vi "OPEN VALVE in Corect Direction.vi"(4 "time after close":u32, 6 "Valve DIR":T1, 7 "changed or first call?":bool, 8 "error in (no error)":errorcluster, 11 "Stand in":refnum<class "Stand.lvclass">) -> (0 "error out":errorcluster, 2 "Done":bool, 3 "Stand out":refnum<class "Stand.lvclass">)   [LabVIEW 2019, in "Stand.lvclass"]
uses:
  Stand.lvclass
  C:/Users/ANENKOV_V1/Desktop/src/Device_class/Device.lvclass
  Valve DIR.ctl
  Device_class/Device.lvclass/Device.ctl
  FPGA/TypeDef/DO index.ctl
  DoValve.vi/e7d2c9dc-ba67-4685-b926-bcce34aa2778.vi
  DoValve.vi/628819af-fd07-4303-9780-3ddd467101db.vi
  Const All Valve.vi
  FPGA_API_class/FPGA API.lvclass
  Device_class/Device.lvclass
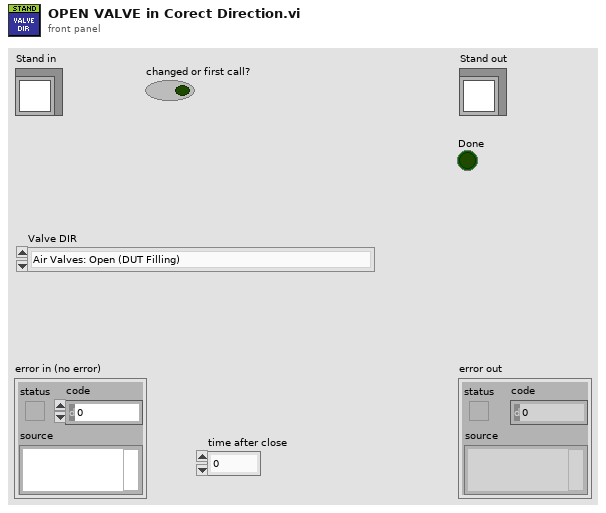
[diagram p1: front panel]
types:
  T1 = typedef "Valve DIR.ctl" = enum16{"Air Valves: Open (DUT Filling)", "Air Valves: Open (Chamber Filling)", "Air Valves: Open (Pump Pressure DUT)", "Air Valves: Open (Pump Pressure Chamber)", "Air Valves: Open (Haskel Pressure DUT)", "Air Valves: Open (Haskel Pressure Chamber)", "Air Valves: Open (Slow Release DUT)", "Air Valves: Open (Slow Release Chamber)", "Air Valves: Open (Fast Release DUT)", "Air Valves: Open (Fast Release Chamber)", "Air Valves: Open (Emergency Release DUT and Chamber)", "Air Valves: Leak Hi (Chamber)", "Air Valves: Leak Hi (DUT)", "Air Valves: Backpressure (Chamber)", "Air Valves: Backpressure (DUT)", "Air Valves: Fully Closed", "Air Valves: Open 33.7"}
  T2 = typedef "DO index.ctl" = u8
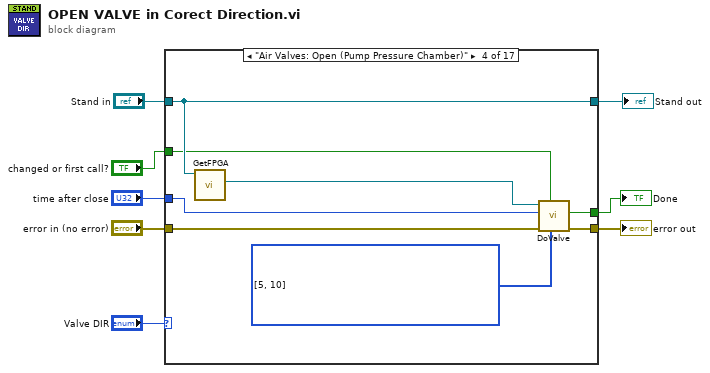
[diagram p0: block diagram]
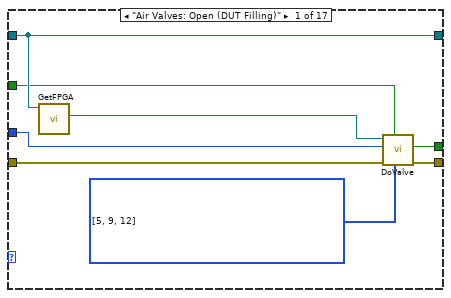
[diagram p2: hidden frame]
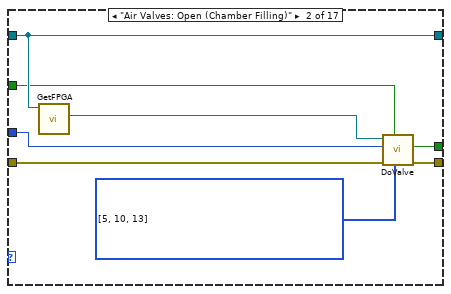
[diagram p3: hidden frame]
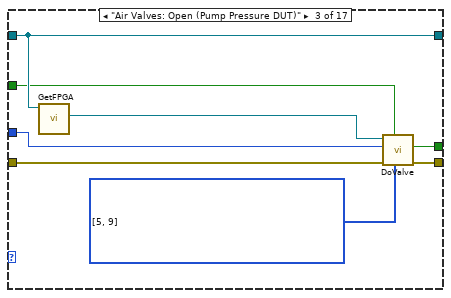
[diagram p4: hidden frame]
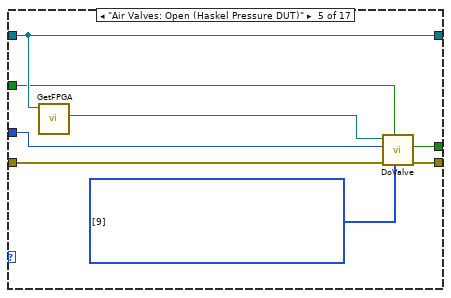
[diagram p5: hidden frame]
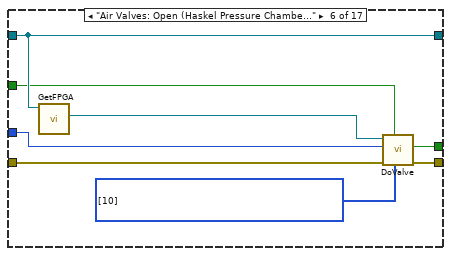
[diagram p6: hidden frame]
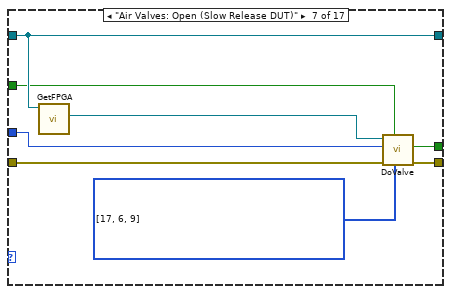
[diagram p7: hidden frame]
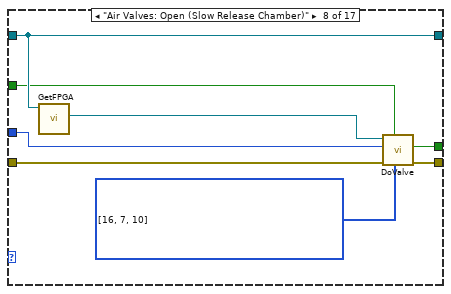
[diagram p8: hidden frame]
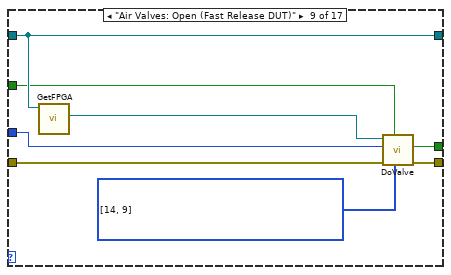
[diagram p9: hidden frame]
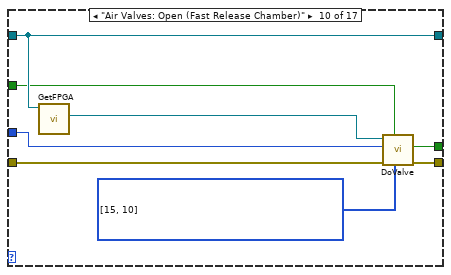
[diagram p10: hidden frame]
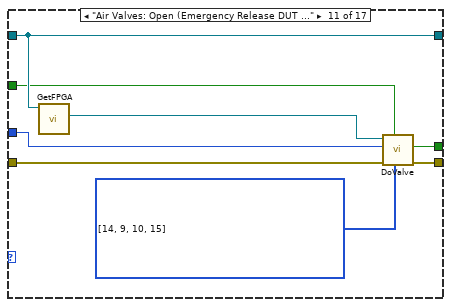
[diagram p11: hidden frame]
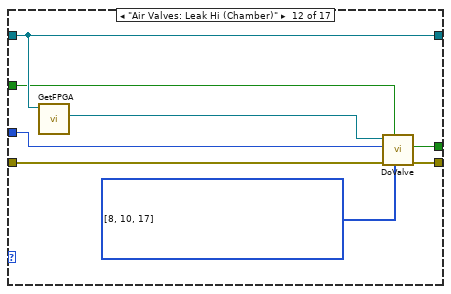
[diagram p12: hidden frame]
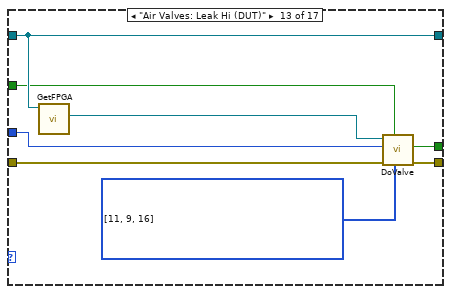
[diagram p13: hidden frame]
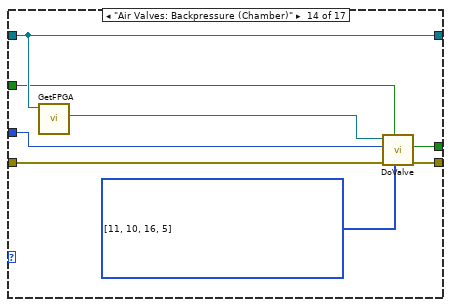
[diagram p14: hidden frame]
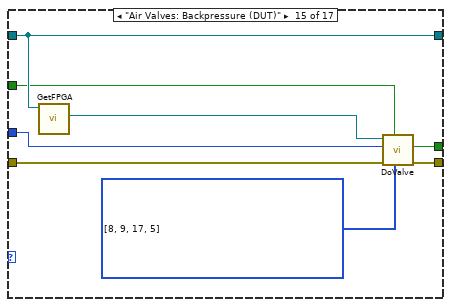
[diagram p15: hidden frame]
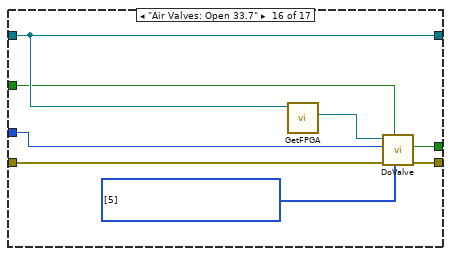
[diagram p16: hidden frame]
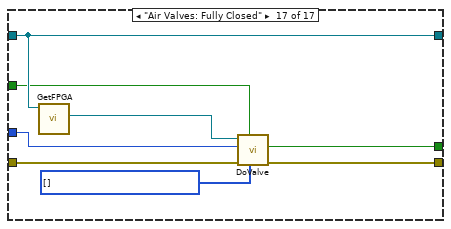
[diagram p17: hidden frame]
diagram:
  n1 = case shown="\"Air Valves: Open (Pump Pressure Chamber)\"" "Valve DIR" {
    tunnel: [w16 w24 w32 w40 w48 w56 w64 w72 w80 w88 w96 w104 w112 w120 w128 w136 w144] -> w3
    tunnel: "Stand in" -> [w16 w24 w32 w40 w48 w56 w64 w72 w80 w88 w96 w104 w112 w120 w128 w136 w144]
    tunnel: [w12 w21 w29 w37 w45 w53 w61 w69 w77 w85 w93 w101 w109 w117 w125 w133 w141] -> w8
    tunnel: "error in (no error)" -> [w14 w22 w30 w38 w46 w54 w62 w70 w78 w86 w94 w102 w110 w118 w126 w134 w142]
    tunnel: [w10 w18 w26 w34 w42 w50 w58 w66 w74 w83 w90 w98 w106 w114 w122 w130 w138] -> w2
    tunnel: "changed or first call?" -> [w11 w19 w27 w35 w43 w51 w59 w67 w75 w82 w91 w99 w107 w115 w123 w131 w139]
    tunnel: "time after close" -> [w9 w17 w25 w33 w41 w49 w57 w65 w73 w81 w89 w97 w105 w113 w121 w129 w137]
    frame "Air Valves: Open (DUT Filling)" {
      w13 = T2[] [5, 9, 12] items=["DO 0 [KP1] [M12]", "DO 1 [ON KP2] [M21]", "DO 2 [ON KP3] [M24]", "DO 3 [WATER Y18.1 [DO3]]", "DO 4 [WATER Y18.2 [DO4]]", "DO 5 [KP6 Y29.1 33.7]", "DO 6 [KP7 Y29.2 33.8]", "DO 7 [KP8 Y29.3 33.9]", "DO 8 [KP9 Y29.4  33.12]", "DO 9 [KP10 Y29.5 33.1]", "DO 10 [KP11 Y29.6 33.2]", "DO 11 [KP12 Y29.7  33.13]", "DO 12 [KP13 Y29.8  33.11]", "DO 13 [KP14 Y29.9 33.10]", "DO 14 [KP15 Y29.10  33.6]", "DO 15 [KP16 Y29.11  33.5]", "DO 16 [KP17 Y29.12  33.4]", "DO 17 [KP18 Y29.13 33.3]", "DO 18 [AIR KP19]", "DO 19 [STEP DRIVE EN KP20]", "DO 20 [KP21 Y44.1 OPEN]", "DO 21 [ KP22 Y44.1 CLOSE]", "DO 22 [ KP23 Y44.2 OPEN]", "DO 23", "DO 24 [STEP DRIVE 1]", "DO 25 [STEP DRIVE 2]"] ("#DO")
      n2 = call "GetFPGA.vi"("Device in"=w16) -> ("FPGA API.lvclass"=w15:refnum<class "FPGA API.lvclass">)  [unwired: 10 in]
      n3 = call "DoValve.vi"("#DO"=w13, "Reset"=w11, "error in (no error)"=w14, "time after close"=w9, "reference in"=w15) -> ("error out"=w12:errorcluster, "Done"=w10:bool)  [unwired: 4 in, 1 out]
    }
    frame "Air Valves: Open (Chamber Filling)" {
      w20 = T2[] [5, 10, 13] items=["DO 0 [KP1] [M12]", "DO 1 [ON KP2] [M21]", "DO 2 [ON KP3] [M24]", "DO 3 [WATER Y18.1 [DO3]]", "DO 4 [WATER Y18.2 [DO4]]", "DO 5 [KP6 Y29.1 33.7]", "DO 6 [KP7 Y29.2 33.8]", "DO 7 [KP8 Y29.3 33.9]", "DO 8 [KP9 Y29.4  33.12]", "DO 9 [KP10 Y29.5 33.1]", "DO 10 [KP11 Y29.6 33.2]", "DO 11 [KP12 Y29.7  33.13]", "DO 12 [KP13 Y29.8  33.11]", "DO 13 [KP14 Y29.9 33.10]", "DO 14 [KP15 Y29.10  33.6]", "DO 15 [KP16 Y29.11  33.5]", "DO 16 [KP17 Y29.12  33.4]", "DO 17 [KP18 Y29.13 33.3]", "DO 18 [AIR KP19]", "DO 19 [STEP DRIVE EN KP20]", "DO 20 [KP21 Y44.1 OPEN]", "DO 21 [ KP22 Y44.1 CLOSE]", "DO 22 [ KP23 Y44.2 OPEN]", "DO 23", "DO 24 [STEP DRIVE 1]", "DO 25 [STEP DRIVE 2]"] ("#DO")
      n4 = call "GetFPGA.vi"("Device in"=w24) -> ("FPGA API.lvclass"=w23:refnum<class "FPGA API.lvclass">)  [unwired: 10 in]
      n5 = call "DoValve.vi"("#DO"=w20, "Reset"=w19, "error in (no error)"=w22, "time after close"=w17, "reference in"=w23) -> ("error out"=w21:errorcluster, "Done"=w18:bool)  [unwired: 4 in, 1 out]
    }
    frame "Air Valves: Open (Pump Pressure DUT)" {
      w28 = T2[] [5, 9] items=["DO 0 [KP1] [M12]", "DO 1 [ON KP2] [M21]", "DO 2 [ON KP3] [M24]", "DO 3 [WATER Y18.1 [DO3]]", "DO 4 [WATER Y18.2 [DO4]]", "DO 5 [KP6 Y29.1 33.7]", "DO 6 [KP7 Y29.2 33.8]", "DO 7 [KP8 Y29.3 33.9]", "DO 8 [KP9 Y29.4  33.12]", "DO 9 [KP10 Y29.5 33.1]", "DO 10 [KP11 Y29.6 33.2]", "DO 11 [KP12 Y29.7  33.13]", "DO 12 [KP13 Y29.8  33.11]", "DO 13 [KP14 Y29.9 33.10]", "DO 14 [KP15 Y29.10  33.6]", "DO 15 [KP16 Y29.11  33.5]", "DO 16 [KP17 Y29.12  33.4]", "DO 17 [KP18 Y29.13 33.3]", "DO 18 [AIR KP19]", "DO 19 [STEP DRIVE EN KP20]", "DO 20 [KP21 Y44.1 OPEN]", "DO 21 [ KP22 Y44.1 CLOSE]", "DO 22 [ KP23 Y44.2 OPEN]", "DO 23", "DO 24 [STEP DRIVE 1]", "DO 25 [STEP DRIVE 2]"] ("#DO")
      n6 = call "GetFPGA.vi"("Device in"=w32) -> ("FPGA API.lvclass"=w31:refnum<class "FPGA API.lvclass">)  [unwired: 10 in]
      n7 = call "DoValve.vi"("#DO"=w28, "Reset"=w27, "error in (no error)"=w30, "time after close"=w25, "reference in"=w31) -> ("error out"=w29:errorcluster, "Done"=w26:bool)  [unwired: 4 in, 1 out]
    }
    frame "Air Valves: Open (Pump Pressure Chamber)" {
      w36 = T2[] [5, 10] items=["DO 0 [KP1] [M12]", "DO 1 [ON KP2] [M21]", "DO 2 [ON KP3] [M24]", "DO 3 [WATER Y18.1 [DO3]]", "DO 4 [WATER Y18.2 [DO4]]", "DO 5 [KP6 Y29.1 33.7]", "DO 6 [KP7 Y29.2 33.8]", "DO 7 [KP8 Y29.3 33.9]", "DO 8 [KP9 Y29.4  33.12]", "DO 9 [KP10 Y29.5 33.1]", "DO 10 [KP11 Y29.6 33.2]", "DO 11 [KP12 Y29.7  33.13]", "DO 12 [KP13 Y29.8  33.11]", "DO 13 [KP14 Y29.9 33.10]", "DO 14 [KP15 Y29.10  33.6]", "DO 15 [KP16 Y29.11  33.5]", "DO 16 [KP17 Y29.12  33.4]", "DO 17 [KP18 Y29.13 33.3]", "DO 18 [AIR KP19]", "DO 19 [STEP DRIVE EN KP20]", "DO 20 [KP21 Y44.1 OPEN]", "DO 21 [ KP22 Y44.1 CLOSE]", "DO 22 [ KP23 Y44.2 OPEN]", "DO 23", "DO 24 [STEP DRIVE 1]", "DO 25 [STEP DRIVE 2]"] ("#DO")
      n8 = call "GetFPGA.vi"("Device in"=w40) -> ("FPGA API.lvclass"=w39:refnum<class "FPGA API.lvclass">)  [unwired: 10 in]
      n9 = call "DoValve.vi"("#DO"=w36, "Reset"=w35, "error in (no error)"=w38, "time after close"=w33, "reference in"=w39) -> ("error out"=w37:errorcluster, "Done"=w34:bool)  [unwired: 4 in, 1 out]
    }
    frame "Air Valves: Open (Haskel Pressure DUT)" {
      w44 = T2[] [9] items=["DO 0 [KP1] [M12]", "DO 1 [ON KP2] [M21]", "DO 2 [ON KP3] [M24]", "DO 3 [WATER Y18.1 [DO3]]", "DO 4 [WATER Y18.2 [DO4]]", "DO 5 [KP6 Y29.1 33.7]", "DO 6 [KP7 Y29.2 33.8]", "DO 7 [KP8 Y29.3 33.9]", "DO 8 [KP9 Y29.4  33.12]", "DO 9 [KP10 Y29.5 33.1]", "DO 10 [KP11 Y29.6 33.2]", "DO 11 [KP12 Y29.7  33.13]", "DO 12 [KP13 Y29.8  33.11]", "DO 13 [KP14 Y29.9 33.10]", "DO 14 [KP15 Y29.10  33.6]", "DO 15 [KP16 Y29.11  33.5]", "DO 16 [KP17 Y29.12  33.4]", "DO 17 [KP18 Y29.13 33.3]", "DO 18 [AIR KP19]", "DO 19 [STEP DRIVE EN KP20]", "DO 20 [KP21 Y44.1 OPEN]", "DO 21 [ KP22 Y44.1 CLOSE]", "DO 22 [ KP23 Y44.2 OPEN]", "DO 23", "DO 24 [STEP DRIVE 1]", "DO 25 [STEP DRIVE 2]"] ("#DO")
      n10 = call "GetFPGA.vi"("Device in"=w48) -> ("FPGA API.lvclass"=w47:refnum<class "FPGA API.lvclass">)  [unwired: 10 in]
      n11 = call "DoValve.vi"("#DO"=w44, "Reset"=w43, "error in (no error)"=w46, "time after close"=w41, "reference in"=w47) -> ("error out"=w45:errorcluster, "Done"=w42:bool)  [unwired: 4 in, 1 out]
    }
    frame "Air Valves: Open (Haskel Pressure Chamber)" {
      w52 = T2[] [10] items=["DO 0 [KP1] [M12]", "DO 1 [ON KP2] [M21]", "DO 2 [ON KP3] [M24]", "DO 3 [WATER Y18.1 [DO3]]", "DO 4 [WATER Y18.2 [DO4]]", "DO 5 [KP6 Y29.1 33.7]", "DO 6 [KP7 Y29.2 33.8]", "DO 7 [KP8 Y29.3 33.9]", "DO 8 [KP9 Y29.4  33.12]", "DO 9 [KP10 Y29.5 33.1]", "DO 10 [KP11 Y29.6 33.2]", "DO 11 [KP12 Y29.7  33.13]", "DO 12 [KP13 Y29.8  33.11]", "DO 13 [KP14 Y29.9 33.10]", "DO 14 [KP15 Y29.10  33.6]", "DO 15 [KP16 Y29.11  33.5]", "DO 16 [KP17 Y29.12  33.4]", "DO 17 [KP18 Y29.13 33.3]", "DO 18 [AIR KP19]", "DO 19 [STEP DRIVE EN KP20]", "DO 20 [KP21 Y44.1 OPEN]", "DO 21 [ KP22 Y44.1 CLOSE]", "DO 22 [ KP23 Y44.2 OPEN]", "DO 23", "DO 24 [STEP DRIVE 1]", "DO 25 [STEP DRIVE 2]"] ("#DO")
      n12 = call "GetFPGA.vi"("Device in"=w56) -> ("FPGA API.lvclass"=w55:refnum<class "FPGA API.lvclass">)  [unwired: 10 in]
      n13 = call "DoValve.vi"("#DO"=w52, "Reset"=w51, "error in (no error)"=w54, "time after close"=w49, "reference in"=w55) -> ("error out"=w53:errorcluster, "Done"=w50:bool)  [unwired: 4 in, 1 out]
    }
    frame "Air Valves: Open (Slow Release DUT)" {
      w60 = T2[] [17, 6, 9] items=["DO 0 [KP1] [M12]", "DO 1 [ON KP2] [M21]", "DO 2 [ON KP3] [M24]", "DO 3 [WATER Y18.1 [DO3]]", "DO 4 [WATER Y18.2 [DO4]]", "DO 5 [KP6 Y29.1 33.7]", "DO 6 [KP7 Y29.2 33.8]", "DO 7 [KP8 Y29.3 33.9]", "DO 8 [KP9 Y29.4  33.12]", "DO 9 [KP10 Y29.5 33.1]", "DO 10 [KP11 Y29.6 33.2]", "DO 11 [KP12 Y29.7  33.13]", "DO 12 [KP13 Y29.8  33.11]", "DO 13 [KP14 Y29.9 33.10]", "DO 14 [KP15 Y29.10  33.6]", "DO 15 [KP16 Y29.11  33.5]", "DO 16 [KP17 Y29.12  33.4]", "DO 17 [KP18 Y29.13 33.3]", "DO 18 [AIR KP19]", "DO 19 [STEP DRIVE EN KP20]", "DO 20 [KP21 Y44.1 OPEN]", "DO 21 [ KP22 Y44.1 CLOSE]", "DO 22 [ KP23 Y44.2 OPEN]", "DO 23", "DO 24 [STEP DRIVE 1]", "DO 25 [STEP DRIVE 2]"] ("#DO")
      n14 = call "GetFPGA.vi"("Device in"=w64) -> ("FPGA API.lvclass"=w63:refnum<class "FPGA API.lvclass">)  [unwired: 10 in]
      n15 = call "DoValve.vi"("#DO"=w60, "Reset"=w59, "error in (no error)"=w62, "time after close"=w57, "reference in"=w63) -> ("error out"=w61:errorcluster, "Done"=w58:bool)  [unwired: 4 in, 1 out]
    }
    frame "Air Valves: Open (Slow Release Chamber)" {
      w68 = T2[] [16, 7, 10] items=["DO 0 [KP1] [M12]", "DO 1 [ON KP2] [M21]", "DO 2 [ON KP3] [M24]", "DO 3 [WATER Y18.1 [DO3]]", "DO 4 [WATER Y18.2 [DO4]]", "DO 5 [KP6 Y29.1 33.7]", "DO 6 [KP7 Y29.2 33.8]", "DO 7 [KP8 Y29.3 33.9]", "DO 8 [KP9 Y29.4  33.12]", "DO 9 [KP10 Y29.5 33.1]", "DO 10 [KP11 Y29.6 33.2]", "DO 11 [KP12 Y29.7  33.13]", "DO 12 [KP13 Y29.8  33.11]", "DO 13 [KP14 Y29.9 33.10]", "DO 14 [KP15 Y29.10  33.6]", "DO 15 [KP16 Y29.11  33.5]", "DO 16 [KP17 Y29.12  33.4]", "DO 17 [KP18 Y29.13 33.3]", "DO 18 [AIR KP19]", "DO 19 [STEP DRIVE EN KP20]", "DO 20 [KP21 Y44.1 OPEN]", "DO 21 [ KP22 Y44.1 CLOSE]", "DO 22 [ KP23 Y44.2 OPEN]", "DO 23", "DO 24 [STEP DRIVE 1]", "DO 25 [STEP DRIVE 2]"] ("#DO")
      n16 = call "GetFPGA.vi"("Device in"=w72) -> ("FPGA API.lvclass"=w71:refnum<class "FPGA API.lvclass">)  [unwired: 10 in]
      n17 = call "DoValve.vi"("#DO"=w68, "Reset"=w67, "error in (no error)"=w70, "time after close"=w65, "reference in"=w71) -> ("error out"=w69:errorcluster, "Done"=w66:bool)  [unwired: 4 in, 1 out]
    }
    frame "Air Valves: Open (Fast Release DUT)" {
      w76 = T2[] [14, 9] items=["DO 0 [KP1] [M12]", "DO 1 [ON KP2] [M21]", "DO 2 [ON KP3] [M24]", "DO 3 [WATER Y18.1 [DO3]]", "DO 4 [WATER Y18.2 [DO4]]", "DO 5 [KP6 Y29.1 33.7]", "DO 6 [KP7 Y29.2 33.8]", "DO 7 [KP8 Y29.3 33.9]", "DO 8 [KP9 Y29.4  33.12]", "DO 9 [KP10 Y29.5 33.1]", "DO 10 [KP11 Y29.6 33.2]", "DO 11 [KP12 Y29.7  33.13]", "DO 12 [KP13 Y29.8  33.11]", "DO 13 [KP14 Y29.9 33.10]", "DO 14 [KP15 Y29.10  33.6]", "DO 15 [KP16 Y29.11  33.5]", "DO 16 [KP17 Y29.12  33.4]", "DO 17 [KP18 Y29.13 33.3]", "DO 18 [AIR KP19]", "DO 19 [STEP DRIVE EN KP20]", "DO 20 [KP21 Y44.1 OPEN]", "DO 21 [ KP22 Y44.1 CLOSE]", "DO 22 [ KP23 Y44.2 OPEN]", "DO 23", "DO 24 [STEP DRIVE 1]", "DO 25 [STEP DRIVE 2]"] ("#DO")
      n18 = call "GetFPGA.vi"("Device in"=w80) -> ("FPGA API.lvclass"=w79:refnum<class "FPGA API.lvclass">)  [unwired: 10 in]
      n19 = call "DoValve.vi"("#DO"=w76, "Reset"=w75, "error in (no error)"=w78, "time after close"=w73, "reference in"=w79) -> ("error out"=w77:errorcluster, "Done"=w74:bool)  [unwired: 4 in, 1 out]
    }
    frame "Air Valves: Open (Fast Release Chamber)" {
      w84 = T2[] [15, 10] items=["DO 0 [KP1] [M12]", "DO 1 [ON KP2] [M21]", "DO 2 [ON KP3] [M24]", "DO 3 [WATER Y18.1 [DO3]]", "DO 4 [WATER Y18.2 [DO4]]", "DO 5 [KP6 Y29.1 33.7]", "DO 6 [KP7 Y29.2 33.8]", "DO 7 [KP8 Y29.3 33.9]", "DO 8 [KP9 Y29.4  33.12]", "DO 9 [KP10 Y29.5 33.1]", "DO 10 [KP11 Y29.6 33.2]", "DO 11 [KP12 Y29.7  33.13]", "DO 12 [KP13 Y29.8  33.11]", "DO 13 [KP14 Y29.9 33.10]", "DO 14 [KP15 Y29.10  33.6]", "DO 15 [KP16 Y29.11  33.5]", "DO 16 [KP17 Y29.12  33.4]", "DO 17 [KP18 Y29.13 33.3]", "DO 18 [AIR KP19]", "DO 19 [STEP DRIVE EN KP20]", "DO 20 [KP21 Y44.1 OPEN]", "DO 21 [ KP22 Y44.1 CLOSE]", "DO 22 [ KP23 Y44.2 OPEN]", "DO 23", "DO 24 [STEP DRIVE 1]", "DO 25 [STEP DRIVE 2]"] ("#DO")
      n20 = call "GetFPGA.vi"("Device in"=w88) -> ("FPGA API.lvclass"=w87:refnum<class "FPGA API.lvclass">)  [unwired: 10 in]
      n21 = call "DoValve.vi"("#DO"=w84, "Reset"=w82, "error in (no error)"=w86, "time after close"=w81, "reference in"=w87) -> ("error out"=w85:errorcluster, "Done"=w83:bool)  [unwired: 4 in, 1 out]
    }
    frame "Air Valves: Open (Emergency Release DUT and Chamber)" {
      w92 = T2[] [14, 9, 10, 15] items=["DO 0 [KP1] [M12]", "DO 1 [ON KP2] [M21]", "DO 2 [ON KP3] [M24]", "DO 3 [WATER Y18.1 [DO3]]", "DO 4 [WATER Y18.2 [DO4]]", "DO 5 [KP6 Y29.1 33.7]", "DO 6 [KP7 Y29.2 33.8]", "DO 7 [KP8 Y29.3 33.9]", "DO 8 [KP9 Y29.4  33.12]", "DO 9 [KP10 Y29.5 33.1]", "DO 10 [KP11 Y29.6 33.2]", "DO 11 [KP12 Y29.7  33.13]", "DO 12 [KP13 Y29.8  33.11]", "DO 13 [KP14 Y29.9 33.10]", "DO 14 [KP15 Y29.10  33.6]", "DO 15 [KP16 Y29.11  33.5]", "DO 16 [KP17 Y29.12  33.4]", "DO 17 [KP18 Y29.13 33.3]", "DO 18 [AIR KP19]", "DO 19 [STEP DRIVE EN KP20]", "DO 20 [KP21 Y44.1 OPEN]", "DO 21 [ KP22 Y44.1 CLOSE]", "DO 22 [ KP23 Y44.2 OPEN]", "DO 23", "DO 24 [STEP DRIVE 1]", "DO 25 [STEP DRIVE 2]"] ("#DO")
      n22 = call "GetFPGA.vi"("Device in"=w96) -> ("FPGA API.lvclass"=w95:refnum<class "FPGA API.lvclass">)  [unwired: 10 in]
      n23 = call "DoValve.vi"("#DO"=w92, "Reset"=w91, "error in (no error)"=w94, "time after close"=w89, "reference in"=w95) -> ("error out"=w93:errorcluster, "Done"=w90:bool)  [unwired: 4 in, 1 out]
    }
    frame "Air Valves: Leak Hi (Chamber)" {
      w100 = T2[] [8, 10, 17] items=["DO 0 [KP1] [M12]", "DO 1 [ON KP2] [M21]", "DO 2 [ON KP3] [M24]", "DO 3 [WATER Y18.1 [DO3]]", "DO 4 [WATER Y18.2 [DO4]]", "DO 5 [KP6 Y29.1 33.7]", "DO 6 [KP7 Y29.2 33.8]", "DO 7 [KP8 Y29.3 33.9]", "DO 8 [KP9 Y29.4  33.12]", "DO 9 [KP10 Y29.5 33.1]", "DO 10 [KP11 Y29.6 33.2]", "DO 11 [KP12 Y29.7  33.13]", "DO 12 [KP13 Y29.8  33.11]", "DO 13 [KP14 Y29.9 33.10]", "DO 14 [KP15 Y29.10  33.6]", "DO 15 [KP16 Y29.11  33.5]", "DO 16 [KP17 Y29.12  33.4]", "DO 17 [KP18 Y29.13 33.3]", "DO 18 [AIR KP19]", "DO 19 [STEP DRIVE EN KP20]", "DO 20 [KP21 Y44.1 OPEN]", "DO 21 [ KP22 Y44.1 CLOSE]", "DO 22 [ KP23 Y44.2 OPEN]", "DO 23", "DO 24 [STEP DRIVE 1]", "DO 25 [STEP DRIVE 2]"] ("#DO")
      n24 = call "GetFPGA.vi"("Device in"=w104) -> ("FPGA API.lvclass"=w103:refnum<class "FPGA API.lvclass">)  [unwired: 10 in]
      n25 = call "DoValve.vi"("#DO"=w100, "Reset"=w99, "error in (no error)"=w102, "time after close"=w97, "reference in"=w103) -> ("error out"=w101:errorcluster, "Done"=w98:bool)  [unwired: 4 in, 1 out]
    }
    frame "Air Valves: Leak Hi (DUT)" {
      w108 = T2[] [11, 9, 16] items=["DO 0 [KP1] [M12]", "DO 1 [ON KP2] [M21]", "DO 2 [ON KP3] [M24]", "DO 3 [WATER Y18.1 [DO3]]", "DO 4 [WATER Y18.2 [DO4]]", "DO 5 [KP6 Y29.1 33.7]", "DO 6 [KP7 Y29.2 33.8]", "DO 7 [KP8 Y29.3 33.9]", "DO 8 [KP9 Y29.4  33.12]", "DO 9 [KP10 Y29.5 33.1]", "DO 10 [KP11 Y29.6 33.2]", "DO 11 [KP12 Y29.7  33.13]", "DO 12 [KP13 Y29.8  33.11]", "DO 13 [KP14 Y29.9 33.10]", "DO 14 [KP15 Y29.10  33.6]", "DO 15 [KP16 Y29.11  33.5]", "DO 16 [KP17 Y29.12  33.4]", "DO 17 [KP18 Y29.13 33.3]", "DO 18 [AIR KP19]", "DO 19 [STEP DRIVE EN KP20]", "DO 20 [KP21 Y44.1 OPEN]", "DO 21 [ KP22 Y44.1 CLOSE]", "DO 22 [ KP23 Y44.2 OPEN]", "DO 23", "DO 24 [STEP DRIVE 1]", "DO 25 [STEP DRIVE 2]"] ("#DO")
      n26 = call "GetFPGA.vi"("Device in"=w112) -> ("FPGA API.lvclass"=w111:refnum<class "FPGA API.lvclass">)  [unwired: 10 in]
      n27 = call "DoValve.vi"("#DO"=w108, "Reset"=w107, "error in (no error)"=w110, "time after close"=w105, "reference in"=w111) -> ("error out"=w109:errorcluster, "Done"=w106:bool)  [unwired: 4 in, 1 out]
    }
    frame "Air Valves: Backpressure (Chamber)" {
      w116 = T2[] [11, 10, 16, 5] items=["DO 0 [KP1] [M12]", "DO 1 [ON KP2] [M21]", "DO 2 [ON KP3] [M24]", "DO 3 [WATER Y18.1 [DO3]]", "DO 4 [WATER Y18.2 [DO4]]", "DO 5 [KP6 Y29.1 33.7]", "DO 6 [KP7 Y29.2 33.8]", "DO 7 [KP8 Y29.3 33.9]", "DO 8 [KP9 Y29.4  33.12]", "DO 9 [KP10 Y29.5 33.1]", "DO 10 [KP11 Y29.6 33.2]", "DO 11 [KP12 Y29.7  33.13]", "DO 12 [KP13 Y29.8  33.11]", "DO 13 [KP14 Y29.9 33.10]", "DO 14 [KP15 Y29.10  33.6]", "DO 15 [KP16 Y29.11  33.5]", "DO 16 [KP17 Y29.12  33.4]", "DO 17 [KP18 Y29.13 33.3]", "DO 18 [AIR KP19]", "DO 19 [STEP DRIVE EN KP20]", "DO 20 [KP21 Y44.1 OPEN]", "DO 21 [ KP22 Y44.1 CLOSE]", "DO 22 [ KP23 Y44.2 OPEN]", "DO 23", "DO 24 [STEP DRIVE 1]", "DO 25 [STEP DRIVE 2]"] ("#DO")
      n28 = call "GetFPGA.vi"("Device in"=w120) -> ("FPGA API.lvclass"=w119:refnum<class "FPGA API.lvclass">)  [unwired: 10 in]
      n29 = call "DoValve.vi"("#DO"=w116, "Reset"=w115, "error in (no error)"=w118, "time after close"=w113, "reference in"=w119) -> ("error out"=w117:errorcluster, "Done"=w114:bool)  [unwired: 4 in, 1 out]
    }
    frame "Air Valves: Backpressure (DUT)" {
      w124 = T2[] [8, 9, 17, 5] items=["DO 0 [KP1] [M12]", "DO 1 [ON KP2] [M21]", "DO 2 [ON KP3] [M24]", "DO 3 [WATER Y18.1 [DO3]]", "DO 4 [WATER Y18.2 [DO4]]", "DO 5 [KP6 Y29.1 33.7]", "DO 6 [KP7 Y29.2 33.8]", "DO 7 [KP8 Y29.3 33.9]", "DO 8 [KP9 Y29.4  33.12]", "DO 9 [KP10 Y29.5 33.1]", "DO 10 [KP11 Y29.6 33.2]", "DO 11 [KP12 Y29.7  33.13]", "DO 12 [KP13 Y29.8  33.11]", "DO 13 [KP14 Y29.9 33.10]", "DO 14 [KP15 Y29.10  33.6]", "DO 15 [KP16 Y29.11  33.5]", "DO 16 [KP17 Y29.12  33.4]", "DO 17 [KP18 Y29.13 33.3]", "DO 18 [AIR KP19]", "DO 19 [STEP DRIVE EN KP20]", "DO 20 [KP21 Y44.1 OPEN]", "DO 21 [ KP22 Y44.1 CLOSE]", "DO 22 [ KP23 Y44.2 OPEN]", "DO 23", "DO 24 [STEP DRIVE 1]", "DO 25 [STEP DRIVE 2]"] ("#DO")
      n30 = call "GetFPGA.vi"("Device in"=w128) -> ("FPGA API.lvclass"=w127:refnum<class "FPGA API.lvclass">)  [unwired: 10 in]
      n31 = call "DoValve.vi"("#DO"=w124, "Reset"=w123, "error in (no error)"=w126, "time after close"=w121, "reference in"=w127) -> ("error out"=w125:errorcluster, "Done"=w122:bool)  [unwired: 4 in, 1 out]
    }
    frame "Air Valves: Open 33.7" {
      w132 = T2[] [5] items=["DO 0 [KP1] [M12]", "DO 1 [ON KP2] [M21]", "DO 2 [ON KP3] [M24]", "DO 3 [WATER Y18.1 [DO3]]", "DO 4 [WATER Y18.2 [DO4]]", "DO 5 [KP6 Y29.1 33.7]", "DO 6 [KP7 Y29.2 33.8]", "DO 7 [KP8 Y29.3 33.9]", "DO 8 [KP9 Y29.4  33.12]", "DO 9 [KP10 Y29.5 33.1]", "DO 10 [KP11 Y29.6 33.2]", "DO 11 [KP12 Y29.7  33.13]", "DO 12 [KP13 Y29.8  33.11]", "DO 13 [KP14 Y29.9 33.10]", "DO 14 [KP15 Y29.10  33.6]", "DO 15 [KP16 Y29.11  33.5]", "DO 16 [KP17 Y29.12  33.4]", "DO 17 [KP18 Y29.13 33.3]", "DO 18 [AIR KP19]", "DO 19 [STEP DRIVE EN KP20]", "DO 20 [KP21 Y44.1 OPEN]", "DO 21 [ KP22 Y44.1 CLOSE]", "DO 22 [ KP23 Y44.2 OPEN]", "DO 23", "DO 24 [STEP DRIVE 1]", "DO 25 [STEP DRIVE 2]"] ("#DO")
      n32 = call "GetFPGA.vi"("Device in"=w136) -> ("FPGA API.lvclass"=w135:refnum<class "FPGA API.lvclass">)  [unwired: 10 in]
      n33 = call "DoValve.vi"("#DO"=w132, "Reset"=w131, "error in (no error)"=w134, "time after close"=w129, "reference in"=w135) -> ("error out"=w133:errorcluster, "Done"=w130:bool)  [unwired: 4 in, 1 out]
    }
    frame "Air Valves: Fully Closed" {
      w140 = T2[] [] items=["DO 0 [KP1] [M12]", "DO 1 [ON KP2] [M21]", "DO 2 [ON KP3] [M24]", "DO 3 [WATER Y18.1 [DO3]]", "DO 4 [WATER Y18.2 [DO4]]", "DO 5 [KP6 Y29.1 33.7]", "DO 6 [KP7 Y29.2 33.8]", "DO 7 [KP8 Y29.3 33.9]", "DO 8 [KP9 Y29.4  33.12]", "DO 9 [KP10 Y29.5 33.1]", "DO 10 [KP11 Y29.6 33.2]", "DO 11 [KP12 Y29.7  33.13]", "DO 12 [KP13 Y29.8  33.11]", "DO 13 [KP14 Y29.9 33.10]", "DO 14 [KP15 Y29.10  33.6]", "DO 15 [KP16 Y29.11  33.5]", "DO 16 [KP17 Y29.12  33.4]", "DO 17 [KP18 Y29.13 33.3]", "DO 18 [AIR KP19]", "DO 19 [STEP DRIVE EN KP20]", "DO 20 [KP21 Y44.1 OPEN]", "DO 21 [ KP22 Y44.1 CLOSE]", "DO 22 [ KP23 Y44.2 OPEN]", "DO 23", "DO 24 [STEP DRIVE 1]", "DO 25 [STEP DRIVE 2]"] ("#DO")
      n34 = call "GetFPGA.vi"("Device in"=w144) -> ("FPGA API.lvclass"=w143:refnum<class "FPGA API.lvclass">)  [unwired: 10 in]
      n35 = call "DoValve.vi"("#DO"=w140, "Reset"=w139, "error in (no error)"=w142, "time after close"=w137, "reference in"=w143) -> ("error out"=w141:errorcluster, "Done"=w138:bool)  [unwired: 4 in, 1 out]
    }
  }
  "error out" <- w8
  "Stand out" <- w3
  "Done" <- w2
